vi "read-EPS-inkscape.vi"() -> ()   [LabVIEW 2014]
doc: "André Romero - 2016\nandretec@ifsc.usp.br\n\nRead EPS files and convert in coordenates"
panel:
  out "Pen":bool[](array[boolean])
  out "Y":dbl[](array[numeric])
  out "X":dbl[](array[numeric])
  in  "file (use dialog)":path=path "C:/Documents and Settings/NI-Vision/Desktop/DecodeX/IFSCdwg.eps"
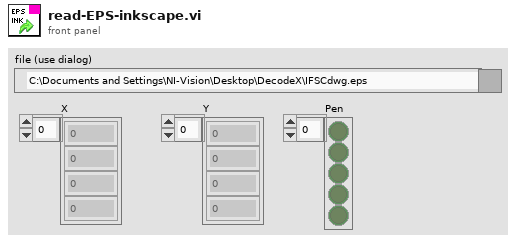
[diagram p1: front panel]
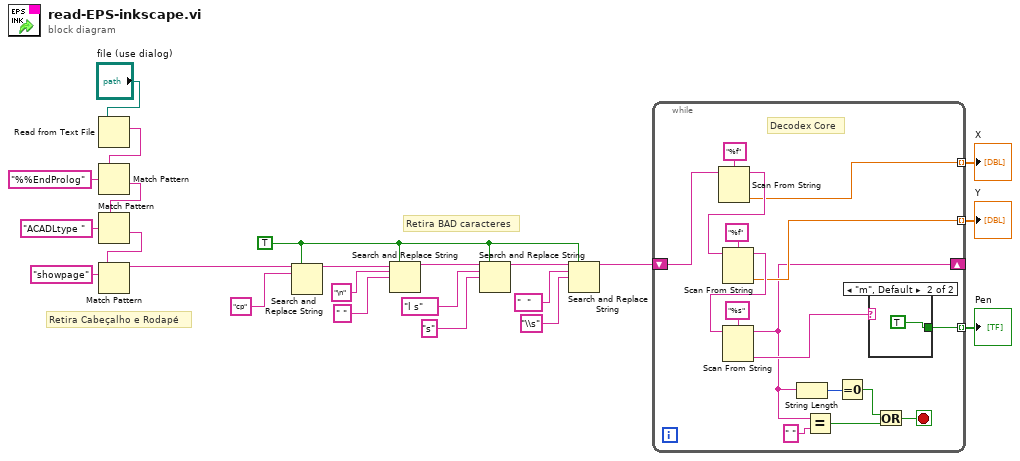
[diagram p0: block diagram]
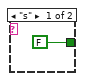
[diagram p2: hidden frame]
diagram:
  w9 = TRUE ("multiline? (F)")
  # "Retira BAD caracteres"
  # "Retira Cabeçalho e Rodapé"
  n1 = Read from Text File(file (use dialog)="file (use dialog)") -> (text=w23:string)  [unwired: 3 in, 3 out]
  n2 = Match Pattern(string=w23, regular expression="%%EndProlog") -> (after substring=w21:string)  [unwired: 1 in, 3 out]
  n3 = Match Pattern(string=w21, regular expression="ACADLtype ") -> (after substring=w18:string)  [unwired: 1 in, 3 out]
  n4 = Match Pattern(string=w18, regular expression="showpage") -> (before substring=w11:string)  [unwired: 1 in, 3 out]
  n5 = Search and Replace String(replace all?=w9, input string=w11, search string="cp") -> (result string=w7:string)  [unwired: 5 in, 3 out]
  n6 = Search and Replace String(replace all?=w9, input string=w7, search string="\n", replace string=" " ("replace string (\"\")")) -> (result string=w6:string)  [unwired: 4 in, 3 out]
  n7 = Search and Replace String(replace all?=w9, input string=w6, search string="l s", replace string="s" ("replace string (\"\")")) -> (result string=w4:string)  [unwired: 4 in, 3 out]
  n8 = Search and Replace String(replace all?=w9, input string=w4, search string="  ", replace string="\\s" ("replace string (\"\")")) -> (result string=w10:string)  [unwired: 4 in, 3 out]
  n9 = while {
    shift-right: [w25] -> _
    shift-left: w10 -> [w34]
    tunnel: [w33] -> w3 mode=indexing
    tunnel: [w32] -> w2 mode=indexing
    tunnel: [w31] -> w1 mode=indexing
    stop <- w28 stop-if-true
    # "Decodex Core"
    n10 = Scan From String(format string="%f", input string=w34) -> (remaining string=w39:string, output 1=w33:dbl)  [unwired: 3 in, 2 out]
    n11 = Scan From String(format string="%f", input string=w39) -> (remaining string=w38:string, output 1=w32:dbl)  [unwired: 3 in, 2 out]
    n12 = Scan From String(format string="%s", input string=w38) -> (remaining string=w25:string, output 1=w30:string)  [unwired: 3 in, 2 out]
    n13 = String Length(string=w25) -> (length=w29:i32)
    n14 = Equal?(x=w25, y=" ") -> (x = y?=w26:bool)
    n15 = Equal To 0?(x=w29) -> (x = 0?=w27:bool)
    n16 = case shown="\"m\", Default" w30 {
      tunnel: [FALSE TRUE] -> w31
      frame "s" {
      }
      frame "m", Default {
      }
    }
    n17 = Or(x=w27, y=w26) -> (x .or. y?=w28:bool)
  }
  "X" <- w3
  "Y" <- w2
  "Pen" <- w1
